vi "Add Port RTM.vi"(8 "error in":errorcluster, 11 "Node Ptr":T1 format="%.0x") -> (0 "error out":errorcluster)   [LabVIEW 2020, in "AIM ARINC 664 System Explorer.lvlib" / "Implementation.lvlib"]
doc: "This VI runs when the Add Port run-time menu is chosen. It allows the user to create a port with an associated database."
uses:
  Implementation.lvlib
  <vilib>/NI VeriStand/Custom Device API/Custom Device Item Ref.ctl
  Scripting/Constants.vi
  <vilib>/NI VeriStand/Custom Device Tools/Custom Device Utility Library/Custom Device Utility Library.lvlib
  <vilib>/NI VeriStand/Custom Device API/Custom Device API.lvlib
  Scripting/AIM ARINC 664 Scripting.lvlib
panel:
  in  "Baud Rate":u32
  in  "Database":string(combo)
  in  "Port Name":string
  in  "Help":bool
  in  "Cancel":bool
  in  "OK":bool
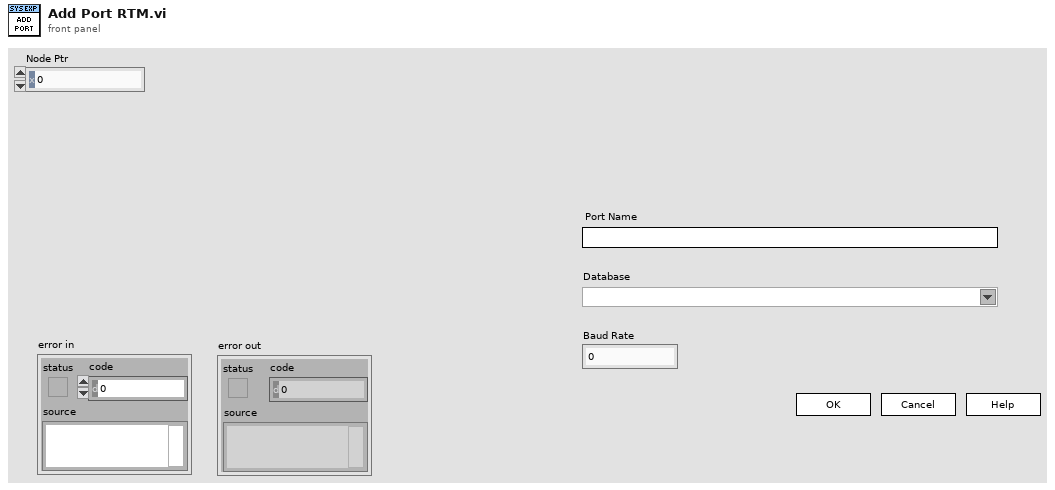
[diagram p1: front panel]
types:
  T1 = typedef "Custom Device API.lvlib/Custom Device Item Ref.ctl" = u64
  T2 = cluster{"Baud Rate":u32, "Port Name":string, "Database Name":string, "Database Path":path, "Databases ref":T1, "Node Ptr":T1}
  T3 = typedef "AIM ARINC 664 System Explorer.lvlib/Implementation.lvlib/Database.ctl" = cluster{"Baud Rate":u64, "Frames":cluster{"Name":string, "ID":i32}[]}
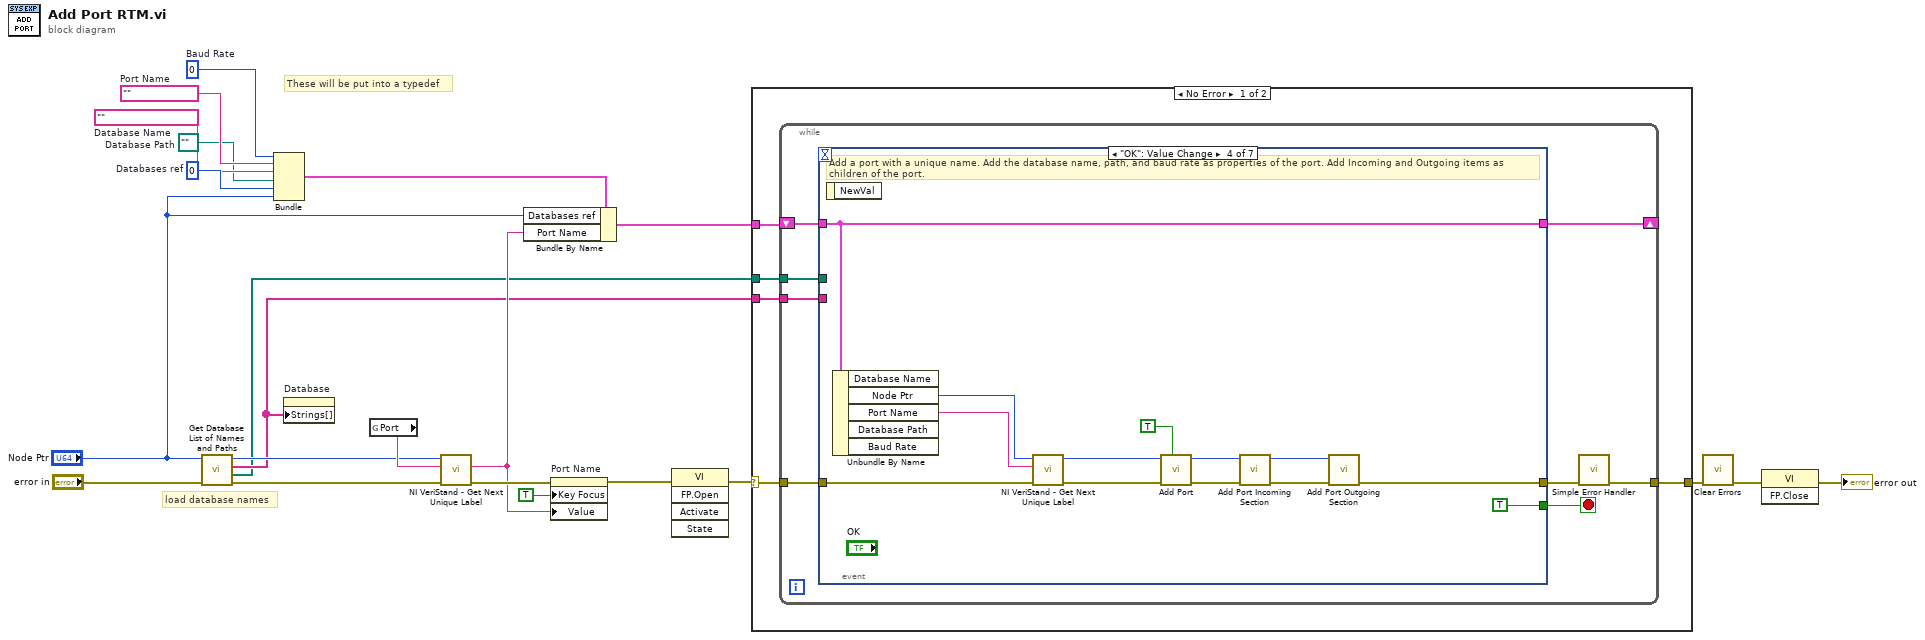
[diagram p0: block diagram]
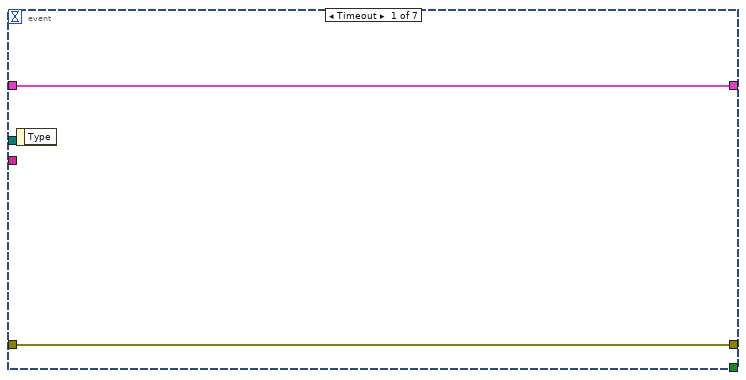
[diagram p2: hidden frame]
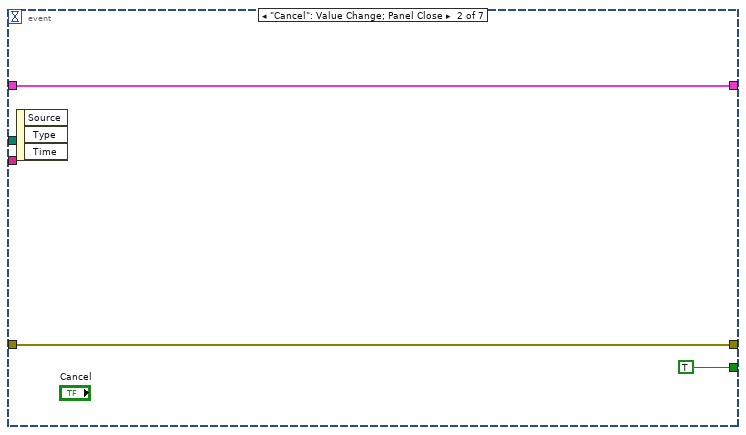
[diagram p3: hidden frame]
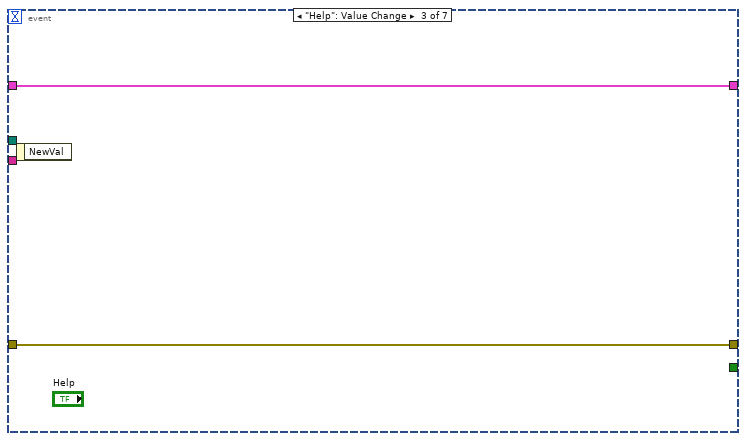
[diagram p4: hidden frame]
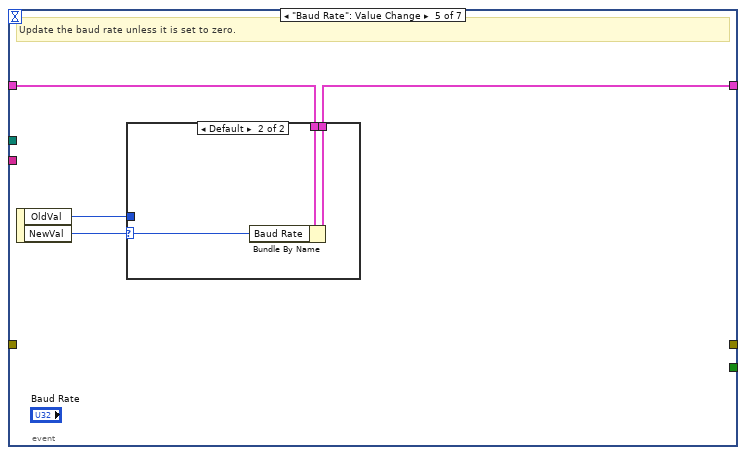
[diagram p5: hidden frame]
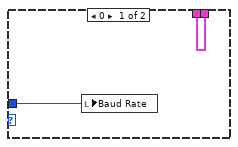
[diagram p6: hidden frame]
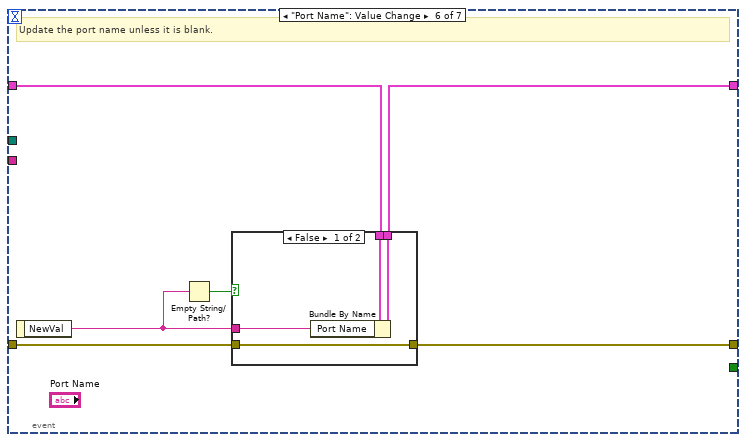
[diagram p7: hidden frame]
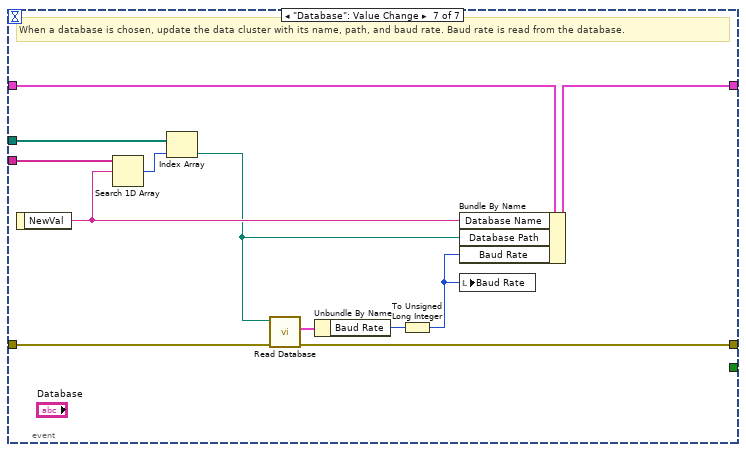
[diagram p9: hidden frame]
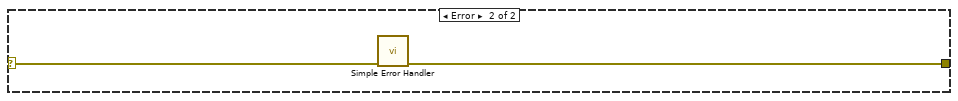
[diagram p10: hidden frame]
diagram:
  w6 = u32 0  # Baud Rate
  w7 = path ""  # Database Path
  w9 = ""  # Database Name
  w12 = T1 0  # Databases ref
  w8 = ""  # Port Name
  # "These will be put into a typedef"
  # "load database names"
  n1 = call "Get Database List of Names and Paths.vi"("error in"="error in", "Databases section Ref"="Node Ptr") -> ("error out"=w4:errorcluster, "Paths"=w1:path[], "Names"=w2:string[], "Databases section Ref out"=w3:T1)  [unwired: 6 in]
  n2 = Bundle("Baud Rate"=w6, "Port Name"=w8, "Database Name"=w9, "Database Path"=w7, "Databases ref"=w12, "Node Ptr"="Node Ptr") -> (w13:T2)  [unwired: 1 in]
  n3 = property on="Database" class="CmbBox"("Strings[]"=w2) -> ()  [unwired: 2 in, 2 out]
  n4 = global read "Constants.vi" "Port"() -> (w14:string)
  n5 = call <vilib>:"NI VeriStand - Get Next Unique Label.vi"("error in (no error)"=w4, "Label"=w14, "Parent Ref in"=w3) -> ("error out"=w15:errorcluster, "Label out"=w11:string)  [unwired: 5 in, 2 out]
  n6 = Bundle By Name(cluster=w13, "Databases ref"="Node Ptr", "Port Name"=w11) -> (w20:T2)
  n7 = property on="Port Name" class="Str"(error in=w15, "Key Focus"=TRUE, "Value"=w11) -> (error out=w19:errorcluster)  [unwired: 1 in, 1 out]
  n8 = invoke class="VI" method="FP.Open"(error in=w19) -> (error out=w18:errorcluster)  [unwired: 4 in, 4 out]
  n9 = case shown="No Error" w18 {
    selector: w18 -> [w27 w90]
    tunnel: [w26 w89] -> w21
    tunnel: w20 -> [w25 _]
    tunnel: w2 -> [w24 _]
    tunnel: w1 -> [w23 _]
    frame No Error {
      n10 = while {
        tunnel: w27 -> [w35]
        tunnel: [w33] -> w26
        shift-right: [w30] -> _
        shift-left: w25 -> [w31]
        tunnel: w24 -> [w29]
        tunnel: w23 -> [w28]
        stop <- w32 stop-if-true
        n11 = event shown="[3] \"OK\": Value Change" {
          selector: _ -> [_ _ _ _ _ _ _]
          dyn-events: _ -> [_ _ _ _ _ _ _]
          timeout: _ -> [_ _ _ _ _ _ _]
          tunnel: [w37 w39 w42 w44 _ w69 w85] -> w34
          tunnel: w35 -> [w37 w39 w42 w54 _ w70 w87]
          tunnel: [_ TRUE ("Discard?") _ TRUE ("Discard?") _ _ _] -> w32
          tunnel: w31 -> [w36 w38 w41 w53 w57 w66 w86]
          tunnel: [w36 w38 w41 w53 w58 w65 w88] -> w30
          tunnel: w29 -> [_ _ _ _ _ _ w80]
          tunnel: w28 -> [_ _ _ _ _ _ w81]
          event Timeout {
            n12 = event-data() -> ()  [unwired: 1 in, 1 out]
          }
          event "Cancel": Value Change; Panel Close {
            n13 = event-data() -> ()  [unwired: 1 in, 3 out]
          }
          event "Help": Value Change {
            n14 = event-data() -> ()  [unwired: 1 in, 1 out]
          }
          event "OK": Value Change {
            # "Add a port with a unique name. Add the database name, path, and baud rate as properties of the port. Add Incoming and Outgoing items as children of the port."
            n15 = event-data() -> ()  [unwired: 1 in, 1 out]
            n16 = Unbundle By Name(w53) -> ("Node Ptr"=w52:T1, "Port Name"=w51:string)  [unwired: 3 out]
            n17 = call <vilib>:"NI VeriStand - Get Next Unique Label.vi"("error in (no error)"=w54, "Label"=w51, "Parent Ref in"=w52) -> ("error out"=w50:errorcluster, "Parent Ref dup"=w49:T1)  [unwired: 5 in, 2 out]
            n18 = call "Add Port.vi"("Highlight? (F)"=TRUE, "error in"=w50, "ports ref"=w49) -> ("error out"=w47:errorcluster, "ports ref out"=w46:T1)  [unwired: 6 in, 1 out]
            n19 = call "Add Port Incoming Section.vi"("error in"=w47, "ports ref"=w46) -> ("error out"=w45:errorcluster, "ports ref out"=w43:T1)  [unwired: 7 in, 1 out]
            n20 = call "Add Port Outgoing Section.vi"("error in"=w45, "ports ref"=w43) -> ("error out"=w44:errorcluster)  [unwired: 7 in, 2 out]
          }
          event "Baud Rate": Value Change {
            # "Update the baud rate unless it is set to zero."
            n21 = event-data() -> ("OldVal"=w56:u32, "NewVal"=w59:u32)  [unwired: 1 in]
            n22 = case shown="Default" w59 {
              selector: w59 -> [_ w62]
              tunnel: w57 -> [w61 w64]
              tunnel: [w61 w63] -> w58
              tunnel: w56 -> [w60 _]
              frame 0 {
                n23 = local write "Baud Rate"(w60) -> ()
              }
              frame Default {
                n24 = Bundle By Name(cluster=w64, "Baud Rate"=w62) -> (w63:T2)
              }
            }
          }
          event "Port Name": Value Change {
            # "Update the port name unless it is blank."
            n25 = event-data() -> ("NewVal"=w67:string)  [unwired: 1 in]
            n26 = Empty String/Path?(string/path=w67) -> (empty?=w68:bool)
            n27 = case shown="False" w68 {
              tunnel: w70 -> [w74 w76]
              tunnel: w67 -> [w72 _]
              tunnel: [w74 w76] -> w69
              tunnel: w66 -> [w73 w75]
              tunnel: [w71 w75] -> w65
              frame False {
                n28 = Bundle By Name(cluster=w73, "Port Name"=w72) -> (w71:T2)
              }
              frame True {
              }
            }
          }
          event "Database": Value Change {
            # "When a database is chosen, update the data cluster with its name, path, and baud rate. Baud rate is read from the database."
            n29 = event-data() -> ("NewVal"=w79:string)  [unwired: 1 in]
            n30 = Search 1D Array(1D array=w80, element=w79) -> (index of element=w82:i32)  [unwired: 1 in]
            n31 = Index Array(array=w81, index=w82) -> (element=w78:path)
            n32 = call "Read Database.vi"("error in"=w87, "Path"=w78) -> ("error out"=w85:errorcluster, "Database"=w84:T3)  [unwired: 8 in]
            n33 = Unbundle By Name(w84) -> ("Baud Rate"=w83:u64)
            n34 = To Unsigned Long Integer(number=w83) -> (unsigned 32bit integer=w77:u32)
            n35 = Bundle By Name(cluster=w86, "Database Name"=w79, "Database Path"=w78, "Baud Rate"=w77) -> (w88:T2)
            n36 = local write "Baud Rate"(w77) -> ()
          }
        }
        n37 = call <vilib>:"Simple Error Handler.vi"("error in (no error)"=w34) -> ("error out"=w33:errorcluster)  [unwired: 4 in, 4 out]
      }
    }
    frame Error {
      n38 = call <vilib>:"Simple Error Handler.vi"("error in (no error)"=w90) -> ("error out"=w89:errorcluster)  [unwired: 4 in, 4 out]
    }
  }
  n39 = call <vilib>:"Clear Errors.vi"("error in (no error)"=w21) -> ("error out"=w17:errorcluster)  [unwired: 5 in, 1 out]
  n40 = invoke class="VI" method="FP.Close"(error in=w17) -> (error out=→"error out":errorcluster)  [unwired: 2 in, 2 out]
